vi "PH_Stepmotor_BaseClass.PC Absolute Move.vi"(0 "i ref in":refnum<vi>, 1 "axis":i32=-1, 3 "Target (Unit)":dbl, 5 "error in (no error)":errorcluster) -> (14 "i ref out":refnum<vi>, 19 "error out":errorcluster)   [LabVIEW 2014, in "PH_Stepmotor_BaseClass.lvlib"]
doc: "This VI stores the target position in own attributes."
uses:
  PH_Stepmotor_BaseClass.lvlib
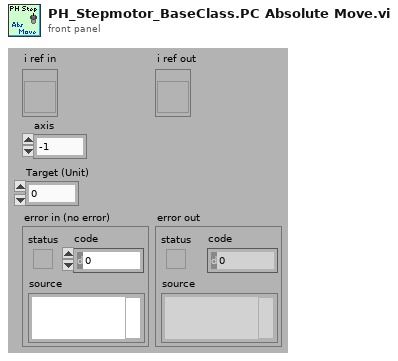
[diagram p1: front panel]
types:
  T1 = typedef "PH_Stepmotor_BaseClass.lvlib/PH_Stepmotor_BaseClass.Axis Attributes.ctl" = cluster{"Settings":T2, "Endswitch?":bool, "DIM Service IDs":T4, "Activity":T5, "Configured?":bool, "Position":cluster{"Current":i32, "Target":i32}, "Position to set":cluster{"New?":bool, "Wanted":i32}, "Stop?":bool, "Reset?":bool, "Move?":bool, "Nothing connected?":bool}
  T2 = typedef "PH_Stepmotor_BaseClass.lvlib/PH_Stepmotor_BaseClass.Axis Settings.ctl" = cluster{"Sign change":bool, "Width":dbl, "Calibration":dbl, "Unit":string, "Motor Type":T3, "Unit Width":string, "Unit CF":string}
  T3 = typedef "PH_Stepmotor_BaseClass.lvlib/PH_Stepmotor_BaseClass.Motor Type.ctl" = enum16{"Unspecific", "OWIS 49.120.2633", "OWIS 49.060.1033", "OWIS 43.040.2558", "Diamond Motion 2200 series", "OWIS 49.120.266B.MV6", "Calorimeter", "Linear Stage 1", "MICOS VT-80", "MICOS VT-80 S", "Standa Rotstage nt0.95A", "PUF RA 320.200", "PUF RA 800.200", "PUF RA 800.400", "PUF RA 400.50", "1324.nn.800.50", "1324.n9c.800.50", "1324.nn.320.200", "1324.nn.400.200", "1324.nn.800.200", "1324.nn.400.50", "1324.8c9c.800.50", "1324.8c9c.400.200"}
  T4 = typedef "PH_Stepmotor_BaseClass.lvlib/PH_Stepmotor_BaseClass.Axis DIM Service IDs.ctl" = cluster{"Settings":i32, "Information":i32}
  T5 = typedef "PH_Stepmotor_BaseClass.lvlib/PH_Stepmotor_BaseClass.Axis Activity.ctl" = enum16{"No Information", "stopped", "running", "Failure", "Alarm", "stopped at backward ES", "stopped at foreward ES"}
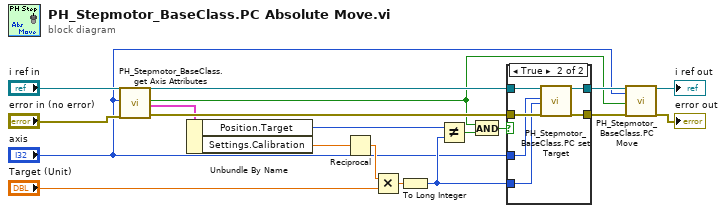
[diagram p0: block diagram]
diagram:
  n1 = call "PH_Stepmotor_BaseClass.get Axis Attributes.vi"("VI in"="i ref in", "Axis"="axis", "error in (no error)"="error in (no error)") -> ("VI out"=w16:refnum<vi>, "Axis found?"=w2:bool, "Axis Attributes"=w15:T1, "error out"=w18:errorcluster)  [unwired: 13 in]
  n2 = Unbundle By Name(w15) -> ("Position.Target"=w10:i32, "Settings.Calibration"=w14:dbl)
  n3 = Reciprocal(x=w14) -> (1/x=w13:dbl)
  n4 = Multiply(x=w13, y="Target (Unit)") -> (x*y=w11:dbl)
  n5 = To Long Integer(number=w11) -> (32bit integer=w9:i32)
  n6 = Not Equal?(x=w10, y=w9) -> (x != y?=w7:bool)
  n7 = And(x=w2, y=w7) -> (x .and. y?=w8:bool)
  n8 = case shown="True" w8 {
    tunnel: [w21 w23] -> w5
    tunnel: [w20 w22] -> w3
    tunnel: w18 -> [w20 w27]
    tunnel: w16 -> [w21 w26]
    tunnel: "axis" -> [_ w24]
    tunnel: w9 -> [_ w25]
    frame False {
    }
    frame True {
      n9 = call "PH_Stepmotor_BaseClass.PC set Target.vi"("VI in"=w26, "axis"=w24, "Targetposition to set"=w25, "error in (no error)"=w27) -> ("VI out"=w23:refnum<vi>, "error out"=w22:errorcluster)  [unwired: 14 in]
    }
  }
  n10 = call "PH_Stepmotor_BaseClass.PC Move.vi"("i ref in"=w5, "axis"="axis", "Move"=w2, "error in (no error)"=w3) -> ("i ref out"=→"i ref out":refnum<vi>, "error out"=→"error out":errorcluster)  [unwired: 14 in]
